vi "Get Tagged Packet Elements from Array.vi"(5 "tagged packet data in":u8[](array[numeric]), 7 "tagged packet offset":u32) -> (4 "packet timestamp":u64, 6 "packet data length (bytes)":u32, 8 "packet data":u8[](array[numeric]), 10 "total tagged packet size (bytes)":u32, 15 "valid packet data?":bool)   [LabVIEW 2023, in "GettingStarted_Common_148X_Host.lvlib"]
uses:
  GettingStarted_Common_148X_Host.lvlib
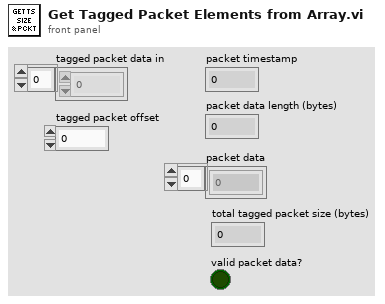
[diagram p1: front panel]
types:
  T1 = enum16{"big-endian, network order", "native, host order", "little-endian"}
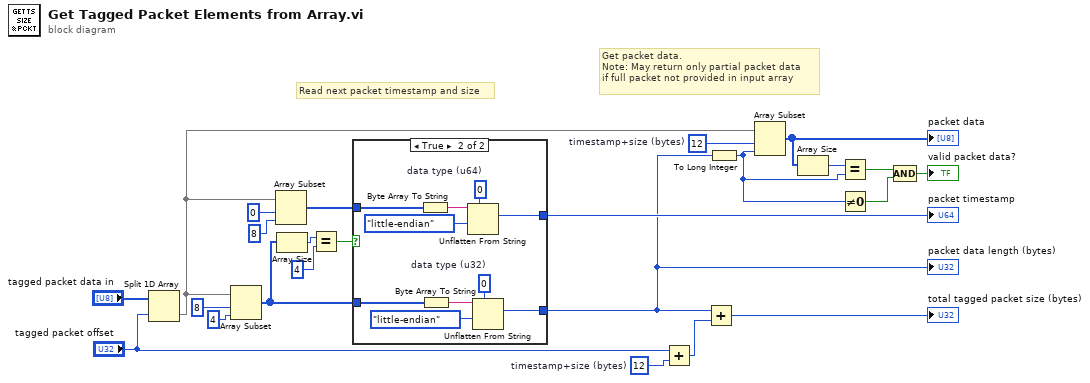
[diagram p0: block diagram]
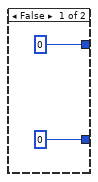
[diagram p2: hidden frame]
diagram:
  w12 = 12  # timestamp+size (bytes)
  w14 = u32 12  # timestamp+size (bytes)
  # "Get packet data.\nNote: May return only partial packet data\nif full packet not provided in input array"
  # "Read next packet timestamp and size"
  n1 = Split 1D Array(array="tagged packet data in", index="tagged packet offset") -> (second subarray=w24:u8[])  [unwired: 1 out]
  n2 = Array Subset(array=w24, index=8, length=4) -> (w23:u8[])
  n3 = Array Subset(array=w24, index=0, length=8 ("index")) -> (w19:u8[])
  n4 = Array Size(array=w23) -> (size(s)=w9:i32)
  n5 = Equal?(x=w9, y=4) -> (x = y?=w4:bool)
  n6 = case shown="True" w4 {
    tunnel: w19 -> [_ w36]
    tunnel: [u64 0 ("data type (u64)") w29] -> w20
    tunnel: [u32 0 ("data type (u32)") w28] -> w11
    tunnel: w23 -> [_ w27]
    frame False {
    }
    frame True {
      w30 = u32 0  # data type (u32)
      w31 = u64 0  # data type (u64)
      n7 = Byte Array To String(unsigned byte array=w36) -> (string=w35:string)
      n8 = Byte Array To String(unsigned byte array=w27) -> (string=w33:string)
      n9 = Unflatten From String(type=w31, binary string=w35, byte order (0:big-endian, network order)=T1."little-endian") -> (value=w29:u64)  [unwired: 2 in, 2 out]
      n10 = Unflatten From String(type=w30, binary string=w33, byte order (0:big-endian, network order)=T1."little-endian") -> (value=w28:u32)  [unwired: 2 in, 2 out]
    }
  }
  "packet data length (bytes)" <- w11
  "packet timestamp" <- w20
  n11 = Add(x="tagged packet offset", y=w14) -> (x+y=w10:u32)
  n12 = Add(x=w11, y=w10) -> (x+y=→"total tagged packet size (bytes)":u32)
  n13 = To Long Integer(number=w11) -> (32bit integer=w2:i32)
  n14 = Array Subset(array=w24, index=w12, length=w2) -> (w13:u8[])
  "packet data" <- w13
  n15 = Array Size(array=w13) -> (size(s)=w7:i32)
  n16 = Equal?(x=w7, y=w2) -> (x = y?=w5:bool)
  n17 = Not Equal To 0?(x=w2) -> (x != 0?=w1:bool)
  n18 = Compound Arithmetic op=AND(w5, w1) -> (→"valid packet data?":bool)
